vi "Latching Relay.vi"(1 "Reset":bool, 2 "Trigger":bool) -> (0 "output":bool)   [LabVIEW 2009]
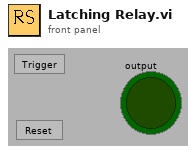
[diagram p1: front panel]
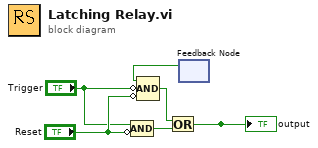
[diagram p0: block diagram]
diagram:
  n1 = Compound Arithmetic op=AND("Trigger", invert "Reset") -> (w6:bool)
  n2 = feedback #1() -> (w1:bool)  [unwired: 1 in]
  n3 = Compound Arithmetic op=AND(w1, invert "Trigger", invert "Reset") -> (w5:bool)
  n4 = Or(x=w5, y=w6) -> (x .or. y?=w3:bool)
  "output" <- w3
